vi "Read Reader IDs.vi"(8 "error in (no error)":errorcluster, 11 "Waveforms (N Ch) in":refnum<class "Waveforms (N Ch).lvclass">) -> (0 "error out":errorcluster, 2 "reader IDs":string[](array[string]), 3 "Waveforms (N Ch) out":refnum<class "Waveforms (N Ch).lvclass">)   [LabVIEW 2017, in "Waveforms (N Ch).lvclass"]
uses:
  <vilib>/addons/_NISVFA/_Shared subVIs/Data Objects/Waveforms (DBL)/Waveforms (N Ch).lvclass
  C:/Program Files (x86)/National Instruments/LabVIEW 2017/vi.lib/addons/_NISVFA/_Shared subVIs/Data Objects/Data/Data.lvclass
  <vilib>/addons/_NISVFA/_Shared subVIs/Data Objects/Data/Data.lvclass/Data.ctl
  <vilib>/addons/_NISVFA/_Shared subVIs/Data Objects/Data/Data.lvclass
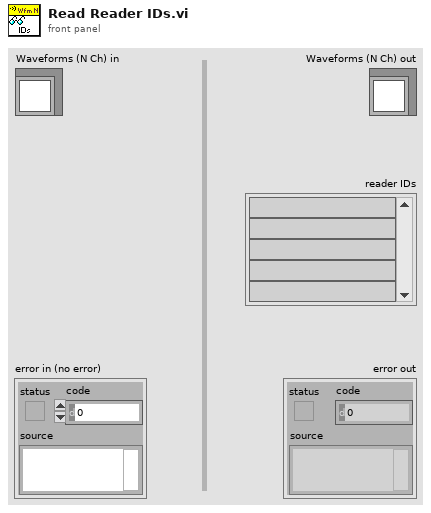
[diagram p1: front panel]
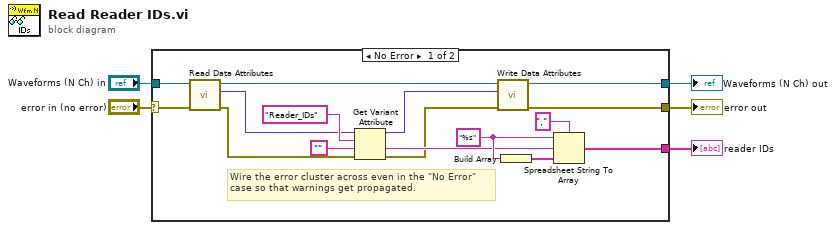
[diagram p0: block diagram]
diagram:
  n1 = case shown="No Error" "error in (no error)" {
    selector: "error in (no error)" -> [w9 w23]
    tunnel: [w6 w23] -> w4
    tunnel: [w11 w22] -> w2
    tunnel: "Waveforms (N Ch) in" -> [w14 w22]
    tunnel: [w15 _] -> w1
    frame No Error {
      w18 = "%s" ("format string")
      # "Wire the error cluster across even in the \"No Error\"\ncase so that warnings get propagated."
      n2 = call <vilib>:"Read Data Attributes.vi"("error in (no error)"=w9, "Data in"=w14) -> ("error out"=w8:errorcluster, "data attributes"=w13:variant, "Data out"=w12:refnum<class "Waveforms (N Ch).lvclass">)  [unwired: 7 in]
      n3 = Get Variant Attribute(Variant=w13, name="Reader_IDs", default value (empty Variant)="" ("name"), error in=w8) -> (duplicate Variant=w10:variant, value=w16:string, error out=w7:errorcluster)  [unwired: 1 out]
      n4 = call <vilib>:"Write Data Attributes.vi"("error in (no error)"=w7, "data attributes"=w10, "Data in"=w12) -> ("error out"=w6:errorcluster, "Data out"=w11:refnum<class "Waveforms (N Ch).lvclass">)  [unwired: 7 in]
      n5 = Build Array(w18) -> (w20:string[])
      n6 = Spreadsheet String To Array(delimiter (Tab)=",", format string=w18, spreadsheet string=w16, array type (2D Dbl)=w20) -> (array=w15:string[])
    }
    frame Error {
    }
  }
  "error out" <- w4
  "Waveforms (N Ch) out" <- w2
  "reader IDs" <- w1
